vi "Test Sequence.vi"(0 "FeedBack Channel":string[](array[string])=["fgdgfvcbc", "vnfhgjkn", "21354682"], 1 "Test Name":string, 2 "Steps":T2(array[cluster]), 3 "DO":T1) -> (6 "Emergency":bool, 7 "Out":i32, 8 "Condition":bool)   [LabVIEW 2015]
uses:
  Data Acquisition/PCI-USB-DAQ/Digital out put.ctl
  Galobal variable_TI.vi
  Project Setup/Globle Variable/GR_Servo.vi
panel:
  out "Channels (Out)":i32[](array[numeric])
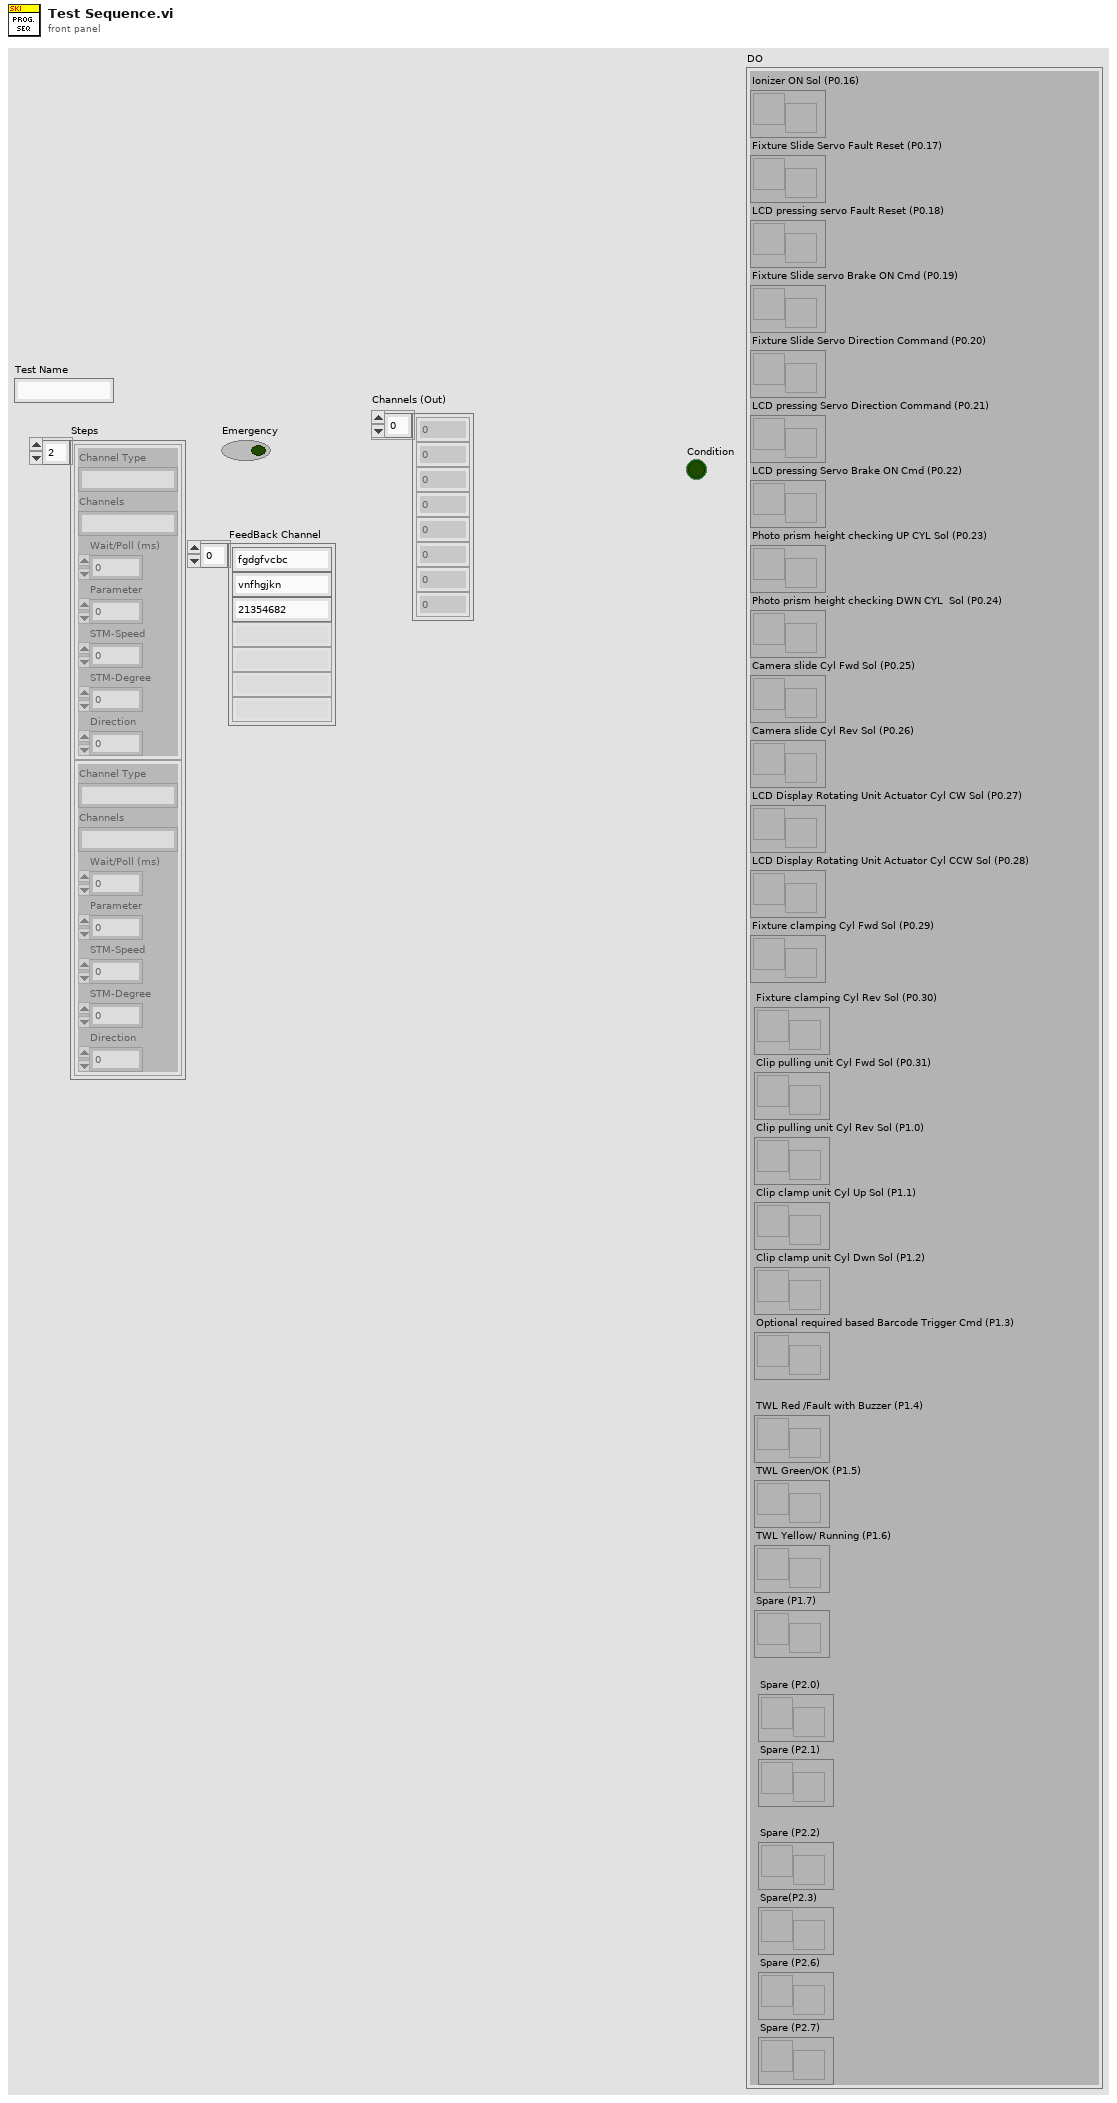
[diagram p1: front panel]
types:
  T1 = typedef "Digital out put.ctl" = cluster{"Ionizer ON Sol (P0.16)":refnum<notifier>, "Fixture Slide Servo Fault Reset (P0.17)":refnum<notifier>, "LCD pressing servo Fault Reset (P0.18)":refnum<notifier>, "Fixture Slide servo Brake ON Cmd (P0.19)":refnum<notifier>, "Fixture Slide Servo Direction Command (P0.20)":refnum<notifier>, "LCD pressing Servo Direction Command (P0.21)":refnum<notifier>, "LCD pressing Servo Brake ON Cmd (P0.22)":refnum<notifier>, "Photo prism height checking UP CYL Sol (P0.23)":refnum<notifier>, "Photo prism height checking DWN CYL  Sol (P0.24)":refnum<notifier>, "Camera slide Cyl Fwd Sol (P0.25)":refnum<notifier>, "Camera slide Cyl Rev Sol (P0.26)":refnum<notifier>, "LCD Display Rotating Unit Actuator Cyl CW Sol (P0.27)":refnum<notifier>, "LCD Display Rotating Unit Actuator Cyl CCW Sol (P0.28)":refnum<notifier>, "Fixture clamping Cyl Fwd Sol (P0.29)":refnum<notifier>, "Fixture clamping Cyl Rev Sol (P0.30)":refnum<notifier>, "Clip pulling unit Cyl Fwd Sol (P0.31)":refnum<notifier>, "Clip pulling unit Cyl Rev Sol (P1.0)":refnum<notifier>, "Clip clamp unit Cyl Up Sol (P1.1)":refnum<notifier>, "Clip clamp unit Cyl Dwn Sol (P1.2)":refnum<notifier>, "Optional required based Barcode Trigger Cmd (P1.3)":refnum<notifier>, "TWL Red /Fault with Buzzer (P1.4)":refnum<notifier>, "TWL Green/OK (P1.5)":refnum<notifier>, "TWL Yellow/ Running (P1.6)":refnum<notifier>, "Spare (P1.7)":refnum<notifier>, "Spare (P2.0)":refnum<notifier>, "Spare (P2.1)":refnum<notifier>, "Spare (P2.2)":refnum<notifier>, "Spare(P2.3)":refnum<notifier>, "Spare (P2.6)":refnum<notifier>, "Spare (P2.7) ":refnum<notifier>}
  T2 = cluster{"Channel Type":string, "Channels":string, "Wait/Poll (ms)":u32, "Parameter":u8, "STM-Speed":i32, "STM-Degree":u32, "Direction":u8}[]
  T3 = cluster{"Emergency":bool, "Air Pressure":bool, "Saftey Sensor":bool, "Slide Servo  fault":bool, "LCD Pressing  Servo  fault":bool}
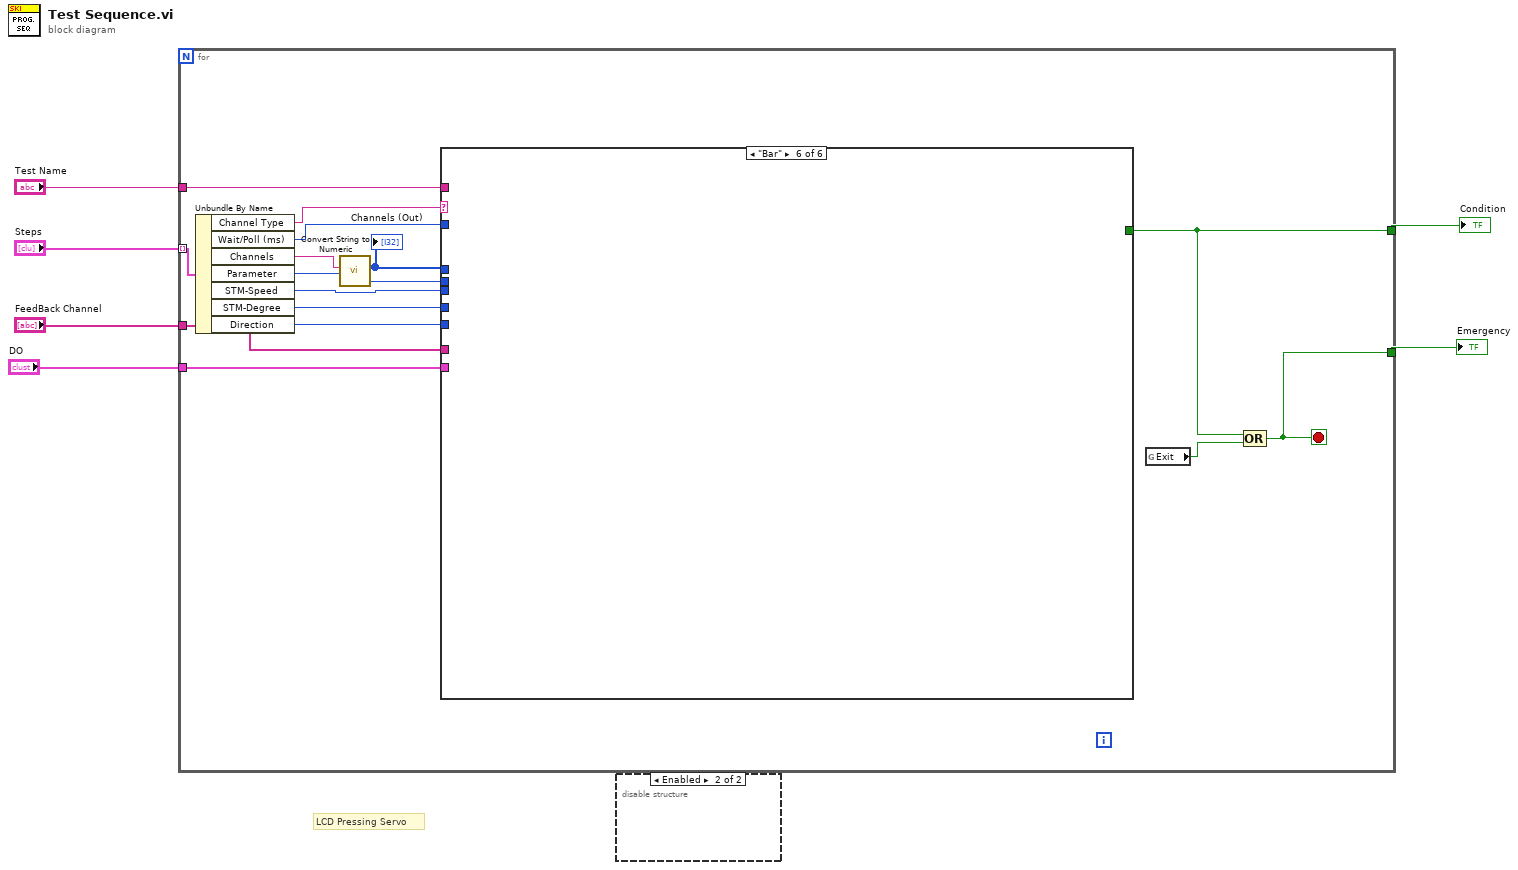
[diagram p0: block diagram]
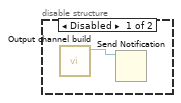
[diagram p2: hidden frame]
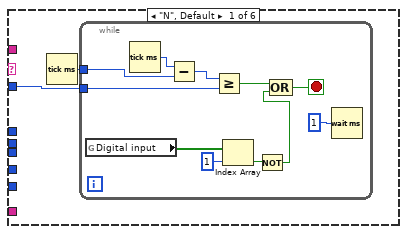
[diagram p3: hidden frame]
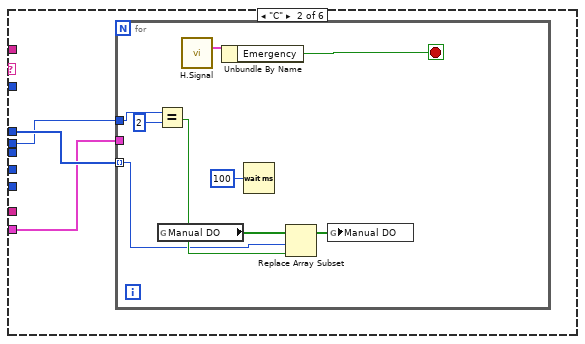
[diagram p4: hidden frame]
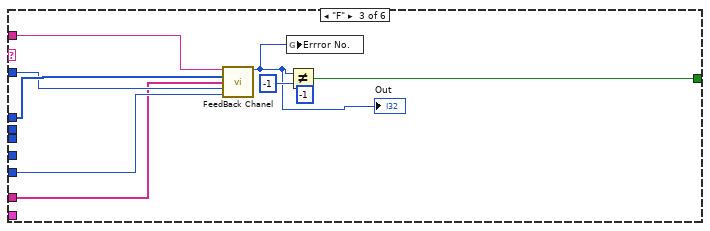
[diagram p5: hidden frame]
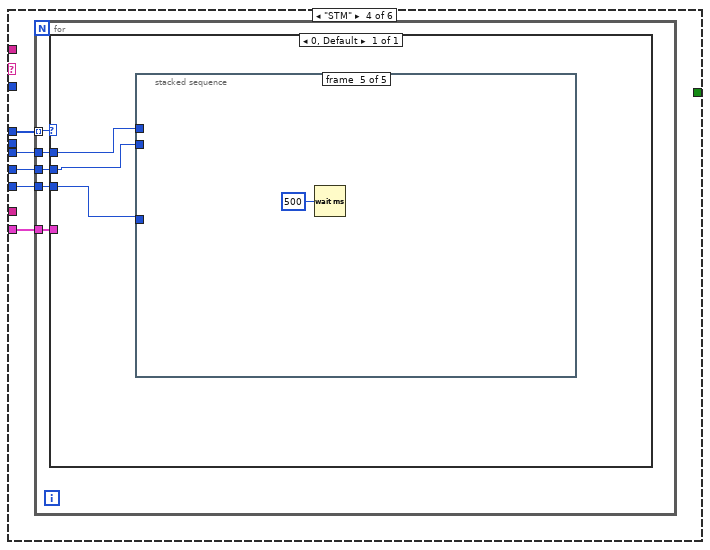
[diagram p6: hidden frame]
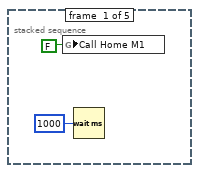
[diagram p7: hidden frame]
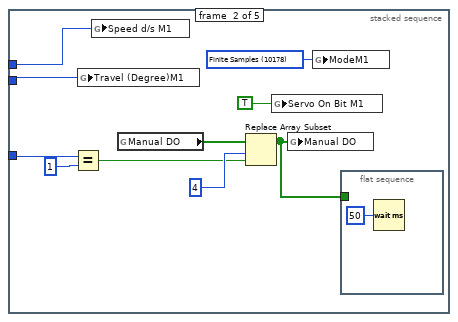
[diagram p8: hidden frame]
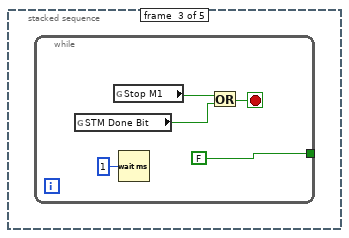
[diagram p9: hidden frame]
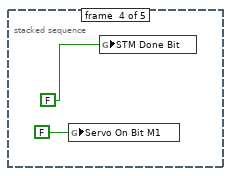
[diagram p10: hidden frame]
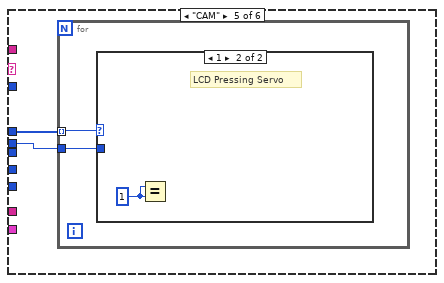
[diagram p11: hidden frame]
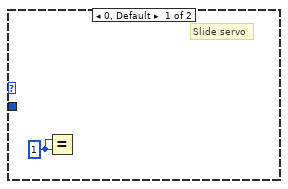
[diagram p12: hidden frame]
diagram:
  # "LCD Pressing Servo"
  n1 = for {
    tunnel: "Steps" -> [w21] mode=indexing
    tunnel: [w13] -> w6
    tunnel: "Test Name" -> [w16]
    tunnel: "FeedBack Channel" -> [w15]
    tunnel: [w12] -> w2
    tunnel: "DO" -> [w11]
    stop <- w13 stop-if-true
    n2 = Unbundle By Name(w21) -> ("Channel Type"=w20:string, "Wait/Poll (ms)"=w19:u32, "Channels"=w18:string, "Parameter"=w7:u8, "STM-Speed"=w9:i32, "STM-Degree"=w8:u32, "Direction"=w10:u8)
    n3 = call "Convert String to Numeric.vi"("Channels (A:B:C:D...) (In)"=w18) -> ("Channels (Out)"=w17:i32[])  [unwired: 9 in, 1 out]
    "Channels (Out)" <- w17
    n4 = case shown="\"Bar\"" w20 {
      tunnel: w19 -> [w22 _ w53 _ _ _]
      tunnel: w17 -> [_ w37 w54 w59 w90 _]
      tunnel: w10 -> [_ _ w52 w58 _ _]
      tunnel: w16 -> [_ _ w51 _ _ _]
      tunnel: w15 -> [_ _ w50 _ _ _]
      tunnel: [_ _ w48 _ _ _] -> w12
      tunnel: w11 -> [_ w36 _ w55 _ _]
      tunnel: w9 -> [_ _ _ w57 _ _]
      tunnel: w8 -> [_ _ _ w56 _ _]
      tunnel: w7 -> [_ w35 _ _ w89 _]
      frame "N", Default {
        n5 = Tick Count (ms)() -> (millisecond timer value=w23:u32)
        n6 = while {
          tunnel: w23 -> [w33]
          tunnel: w22 -> [w28]
          stop <- w29 stop-if-true
          n7 = global read "Galobal variable_TI.vi" "Digital input"() -> (w27:bool[])
          n8 = Tick Count (ms)() -> (millisecond timer value=w34:u32)
          n9 = Subtract(x=w34, y=w33) -> (x-y=w32:u32)
          n10 = Greater Or Equal?(x=w32, y=w28) -> (x >= y?=w30:bool)
          n11 = Index Array(array=w27, index=1) -> (element=w25:bool)
          n12 = Not(x=w25) -> (.not. x?=w24:bool)
          n13 = Compound Arithmetic op=OR(w30, w24) -> (w29:bool)
          n14 = Wait (ms)(milliseconds to wait=u32 1) -> ()  [unwired: 1 out]
        }
      }
      frame "C" {
        n15 = for {
          tunnel: w37 -> [w38] mode=indexing
          tunnel: w35 -> [w46]
          tunnel: w36 -> [_]
          stop <- w42 stop-if-true
          n16 = Equal?(x=w46, y=u8 2) -> (x = y?=w39:bool)
          n17 = global read "Galobal variable_TI.vi" "Manual DO"() -> (w40:bool[])
          n18 = call "H.Signal.vi"() -> ("H.Signal"=w43:T3)  [unwired: 11 in, 4 out]
          n19 = Unbundle By Name(w43) -> ("Emergency"=w42:bool)
          n20 = Wait (ms)(milliseconds to wait=u32 100) -> ()  [unwired: 1 out]
          n21 = Replace Array Subset(array=w40, new element=w39, index=w38) -> (w41:bool[])
          n22 = global write "Galobal variable_TI.vi" "Manual DO"(w41) -> ()
        }
      }
      frame "F" {
        (unwired) -1 ("Out")
        n23 = call "FeedBack Chanel.vi"("Test Name"=w51, "Channels (Int)"=w54, "FeedBack Channel"=w50, "Wait/Poll (ms)"=w53, "Parameter"=w52) -> ("Out"=w47:i32)  [unwired: 7 in, 3 out]
        "Out" <- w47
        n24 = global write "Galobal variable_TI.vi" "Errror No."(w47) -> ()
        n25 = Not Equal?(x=w47, y=-1) -> (x != y?=w48:bool)
      }
      frame "STM" {
        n26 = for {
          tunnel: w59 -> [w64] mode=indexing
          tunnel: w58 -> [w63]
          tunnel: w57 -> [w62]
          tunnel: w56 -> [w61]
          tunnel: w55 -> [w60]
          n27 = case shown="0, Default" w64 {
            tunnel: w63 -> [w65]
            tunnel: w62 -> [w67]
            tunnel: w61 -> [w66]
            tunnel: w60 -> [_]
            frame 0, Default {
              n28 = stacked-sequence {
                tunnel: w66 -> [_ w79 _ _ _]
                tunnel: w65 -> [_ w73 _ _ _]
                tunnel: w67 -> [_ w70 _ _ _]
                frame #0 {
                  n29 = global write "Galobal variable_TI.vi" "Call Home M1"(FALSE ("Call Home M2")) -> ()
                  n30 = Wait (ms)(milliseconds to wait=u32 1000) -> ()  [unwired: 1 out]
                }
                frame #1 {
                  w78 = 10178 items=["Finite Samples"=10178, "Continuous Samples"=10123, "Hardware Timed Single Point"=12522] ("ModeM1")
                  n31 = Equal?(x=w73, y=u8 1) -> (x = y?=w72:bool)
                  n32 = global write "GR_Servo.vi" "Travel (Degree)M1"(w79) -> ()
                  n33 = global write "GR_Servo.vi" "Speed d/s M1"(w70) -> ()
                  n34 = global read "Galobal variable_TI.vi" "Manual DO"() -> (w75:bool[])
                  n35 = Replace Array Subset(array=w75, new element=w72, index=4) -> (w71:bool[])
                  n36 = global write "GR_Servo.vi" "Servo On Bit M1"(TRUE ("Servo On Bit")) -> ()
                  n37 = global write "Galobal variable_TI.vi" "Manual DO"(w71) -> ()
                  n38 = global write "GR_Servo.vi" "ModeM1"(w78) -> ()
                  n39 = flat-sequence {
                    tunnel: w71 -> [_]
                    frame #0 {
                      n40 = Wait (ms)(milliseconds to wait=u32 50) -> ()  [unwired: 1 out]
                    }
                  }
                }
                frame #2 {
                  n41 = while {
                    tunnel: [FALSE] -> _
                    stop <- w82 stop-if-true
                    n42 = global read "Galobal variable_TI.vi" "STM Done Bit"() -> (w81:bool)
                    n43 = global read "Galobal variable_TI.vi" "Stop M1"() -> (w83:bool)
                    n44 = Wait (ms)(milliseconds to wait=u32 1) -> ()  [unwired: 1 out]
                    n45 = Or(x=w83, y=w81) -> (x .or. y?=w82:bool)
                  }
                }
                frame #3 {
                  n46 = global write "GR_Servo.vi" "Servo On Bit M1"(FALSE ("Servo On Bit")) -> ()
                  n47 = global write "Galobal variable_TI.vi" "STM Done Bit"(FALSE ("STM Done Bit LCD Pressing")) -> ()
                }
                frame #4 {
                  n48 = Wait (ms)(milliseconds to wait=u32 500) -> ()  [unwired: 1 out]
                }
              }
            }
          }
        }
      }
      frame "CAM" {
        n49 = for {
          tunnel: w90 -> [w92] mode=indexing
          tunnel: w89 -> [w91]
          n50 = case shown="1" w92 {
            tunnel: w91 -> [_ _]
            frame 0, Default {
              w93 = u8 1 ("y")
              # "Slide servo"
              n51 = Equal?(x=w93, y=w93) -> ()  [unwired: 1 out]
            }
            frame 1 {
              w94 = u8 1 ("y")
              # "LCD Pressing Servo"
              n52 = Equal?(x=w94, y=w94) -> ()  [unwired: 1 out]
            }
          }
        }
      }
      frame "Bar" {
      }
    }
    n53 = global read "Galobal variable_TI.vi" "Exit"() -> (w14:bool)
    n54 = Compound Arithmetic op=OR(w12, w14) -> (w13:bool)
  }
  "Emergency" <- w6
  "Condition" <- w2
  n55 = disable-structure shown="Enabled" {
    frame Disabled {
      n56 = call "Output channel build.vi"() -> ("Output channel"=w95:refnum<notifier>)  [unwired: 11 in]
      n57 = Send Notification(notifier=w95) -> ()  [unwired: 2 in, 2 out]
    }
    frame Enabled {
    }
  }
